vi "FTW-CodeGen-CleanUpWire.vi"(0 "GObject to Traverse":refnum<vi>, 5 "Wire Label":string="@FTW-CodeGen-WireToCleanUp", 11 "error in":errorcluster) -> (4 "GObject to Traverse out":refnum<vi>, 15 "error out":errorcluster)   [LabVIEW 2014]
panel:
  # "Inputs"
  # "Outputs"
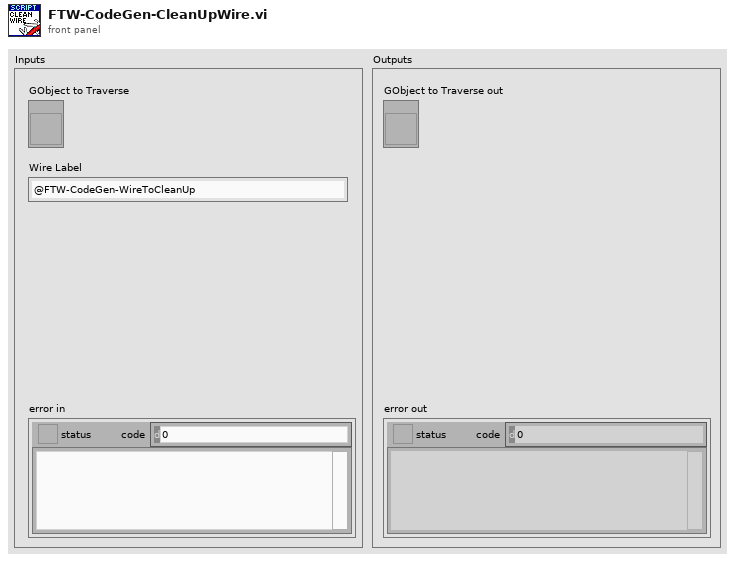
[diagram p1: front panel]
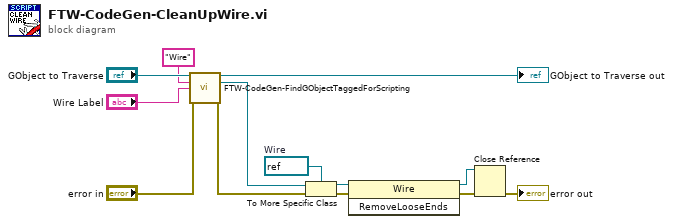
[diagram p0: block diagram]
diagram:
  w8 = refnum<vi> refnum  # Wire
  n1 = call "FTW-CodeGen-FindGObjectTaggedForScripting.vi"("GObject to Traverse"="GObject to Traverse", "Class Name"="Wire", "Label Prefix to uniquely identify node"="Wire Label", "error in"="error in") -> ("GObject to Traverse out"=→"GObject to Traverse out":refnum<vi>, "GObject"=w10:refnum<vi>, "error out"=w2:errorcluster)  [unwired: 9 in]
  n2 = To More Specific Class(target class=w8, reference=w10, error in=w2) -> (specific class reference=w7:refnum<vi>, error out=w1:errorcluster)
  n3 = invoke class="Wire" method="RemoveLooseEnds"(reference=w7, error in=w1) -> (reference out=w5:refnum<vi>, error out=w6:errorcluster)  [unwired: 1 in, 1 out]
  n4 = Close Reference(reference=w5, error in (no error)=w6) -> (error out=→"error out":errorcluster)
